vi "getdata_photosensor.vi"(6 "error in":errorcluster, 7 "Physical Channel":tag="Dev1/ai0", 8 "Number of Samples":i32=100, 9 "Sample Rate":dbl=1000.0, 10 "Min Voltage":dbl=-5.0, 11 "Max Voltage":dbl=5.0) -> (3 "Avg Voltage":dbl=1000.0 format="%0.2f", 4 "error out":errorcluster)   [LabVIEW 2018]
doc: "This VI reads voltage from a specified channel in a DAQ and returns an average value according to the number of configured samples"
uses:
  SupportVIs/DAQmx Read (Analog 1D Wfm NChan NSamp).vi
  SupportVIs/DAQmx Create Channel (AI-Voltage-Basic).vi
  SupportVIs/DAQmx Timing (Sample Clock).vi
  SupportVIs/DAQmx Fill In Error Info.vi
  C:/Program Files/National Instruments/LabVIEW 2018/resource/objmgr/daqmx.rc
panel:
  in  "Stop":bool
  in  "Sample Clock Source":tag="OnboardClock"
  in  "Terminal Configuration":i32(ring)=-1 items=["default"=-1, "RSE"=10083, "NRSE"=10078, "Differential"=10106, "Pseudodifferential"=12529]
  out "Actual Sample Rate":dbl=1000.0 format="%0.2f"
  # "Channel Settings"
  # "Timing Settings"
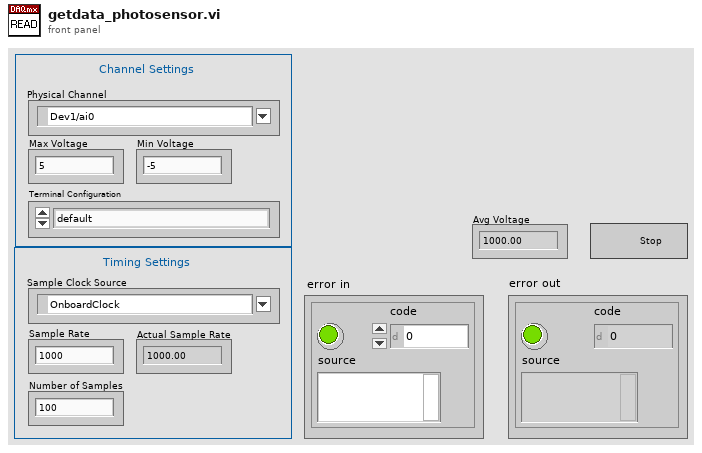
[diagram p1: front panel]
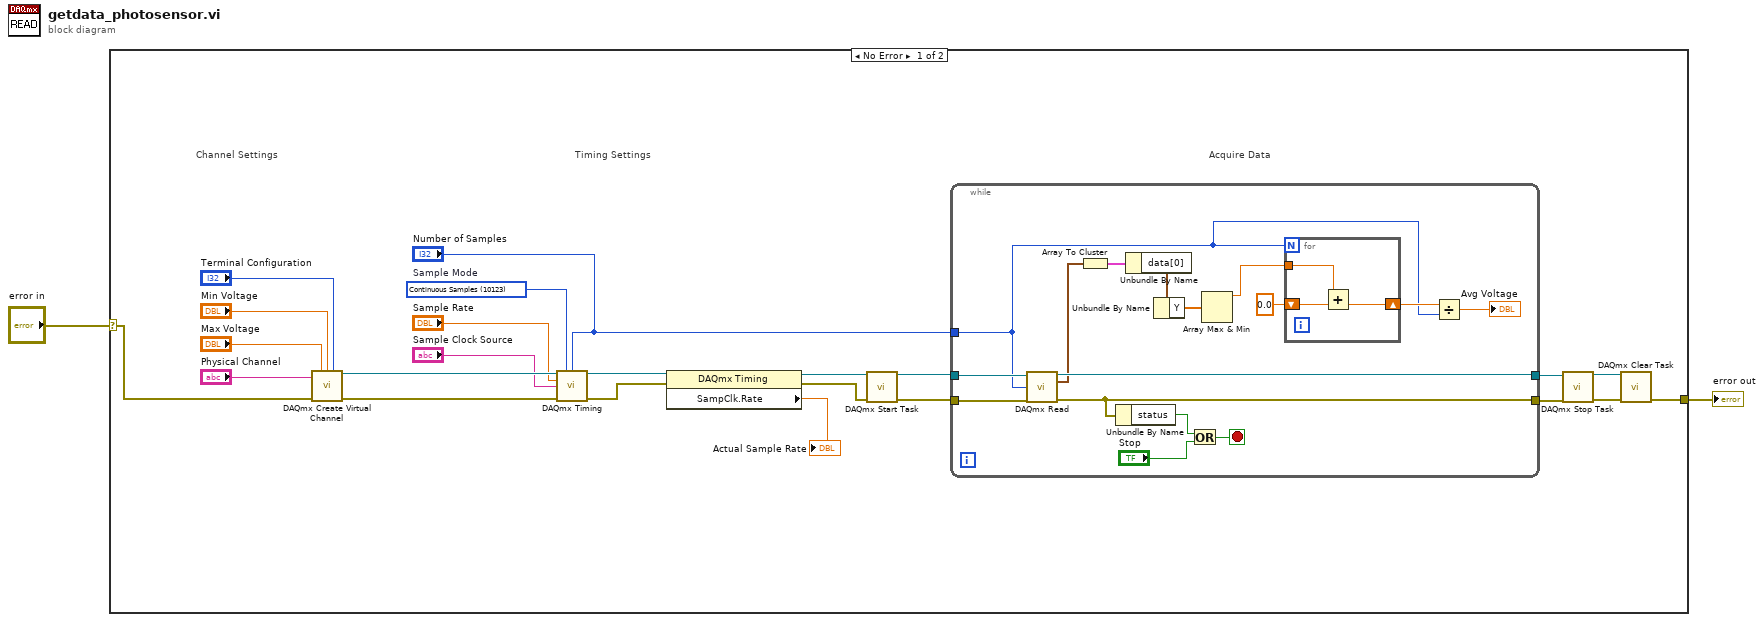
[diagram p0: block diagram]
diagram:
  n1 = case shown="No Error" "error in" {
    selector: "error in" -> [w3 w45]
    tunnel: [w18 w45] -> w2
    frame No Error {
      w23 = 10123 items=["Finite Samples"=10178, "Continuous Samples"=10123, "Hardware Timed Single Point"=12522]  # Sample Mode
      # "Acquire Data"
      # "Timing Settings"
      # "Channel Settings"
      n2 = call-poly "DAQmx Create Virtual Channel.vi"("maximum value"="Max Voltage", "minimum value"="Min Voltage", "input terminal configuration"="Terminal Configuration", "physical channels"="Physical Channel", "error in"=w3) -> ("task out"=w21:refnum<k21>, "error out"=w22:errorcluster)  [unwired: 9 in]
      n3 = call-poly "DAQmx Timing.vi"("task/channels in"=w21, "sample mode"=w23, "samples per channel"="Number of Samples", "rate"="Sample Rate", "source"="Sample Clock Source", "error in"=w22) -> ("task out"=w25:refnum<k21>, "error out"=w24:errorcluster)  [unwired: 8 in]
      n4 = property class="DAQmx Timing"(reference=w25, error in=w24) -> (reference out=w5:refnum<k21>, error out=w4:errorcluster, "SampClk.Rate"=→"Actual Sample Rate":dbl)
      n5 = call "DAQmx Start Task.vi"("task/channels in"=w5, "error in"=w4) -> ("task out"=w20:refnum<k21>, "error out"=w19:errorcluster)  [unwired: 12 in]
      n6 = while {
        tunnel: w20 -> [w41]
        tunnel: w19 -> [w40]
        tunnel: [w39] -> w9
        tunnel: [w37] -> w8
        tunnel: "Number of Samples" -> [w27]
        stop <- w35 stop-if-true
        n7 = call-poly "DAQmx Read.vi"("task/channels in"=w41, "number of samples per channel"=w27, "error in"=w40) -> ("task out"=w39:refnum<k21>, "data"=w34:waveform(dbl)[], "error out"=w37:errorcluster)  [unwired: 10 in]
        n8 = Array To Cluster(array=w34) -> (cluster=w33:cluster{"data[0]":waveform(dbl)})
        n9 = Unbundle By Name(w37) -> ("status"=w36:bool)
        n10 = Unbundle By Name(w33) -> ("data[0]"=w31:waveform(dbl))
        n11 = Unbundle By Name(w31) -> ("Y"=w32:dbl[])
        n12 = Or(x=w36, y="Stop") -> (x .or. y?=w35:bool)
        n13 = Array Max & Min(array=w32) -> (max value=w30:dbl)  [unwired: 3 out]
        n14 = for {
          N: w27 -> [_]
          tunnel: w30 -> [w44]
          shift-right: [w43] -> w28
          shift-left: 0.0 -> [w42]
          n15 = Add(x=w44, y=w42) -> (x+y=w43:dbl)
        }
        n16 = Divide(x=w28, y=w27) -> (x/y=→"Avg Voltage":dbl)
      }
      n17 = call "DAQmx Stop Task.vi"("task/channels in"=w9, "error in"=w8) -> ("task out"=w6:refnum<k21>, "error out"=w7:errorcluster)  [unwired: 12 in]
      n18 = call "DAQmx Clear Task.vi"("task in"=w6, "error in"=w7) -> ("error out"=w18:errorcluster)  [unwired: 13 in]
    }
    frame Error {
    }
  }
  "error out" <- w2
